vi "Scan and Select.vi"(0 "DMM":refnum<visa-resource-name>="COM1", 4 "Charger Selections":enum16{"110", "113", "114", "115", "119", "120"}(ring), 5 "error in":errorcluster) -> (14 "Voltage":dbl format="%0.8f", 19 "error out":errorcluster)   [LabVIEW 2015]
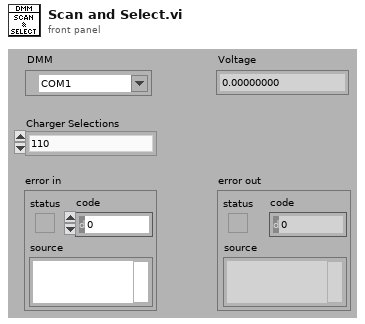
[diagram p1: front panel]
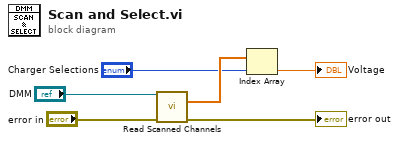
[diagram p0: block diagram]
diagram:
  n1 = call "Read Scanned Channels.vi"("VISA resource name"="DMM", "error in (no error)"="error in") -> ("Measurement Data"=w6:dbl[], "error out"=→"error out":errorcluster)  [unwired: 8 in, 4 out]
  n2 = Index Array(array=w6, index="Charger Selections") -> (element=→"Voltage":dbl)
